vi "Read Actual Position.vi"(4 "error in (no error)":errorcluster, 6 "Axis (1)":i32=1 min=1 max=3, 7 "VISA resource name":refnum<visa-resource-name>) -> (0 "error out":errorcluster, 2 "Position (units)":dbl format="%.6g", 3 "VISA resource name out":refnum<visa-resource-name>)   [LabVIEW 2011, in "Newport ESP301.lvlib"]
doc: "Reads the current position.\nIt returns the instantaneous real position of the specified axis."
uses:
  Newport ESP301.lvlib
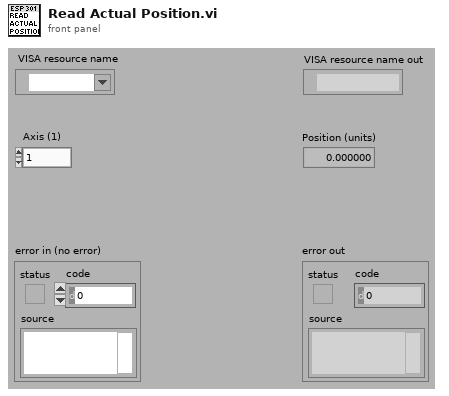
[diagram p1: front panel]
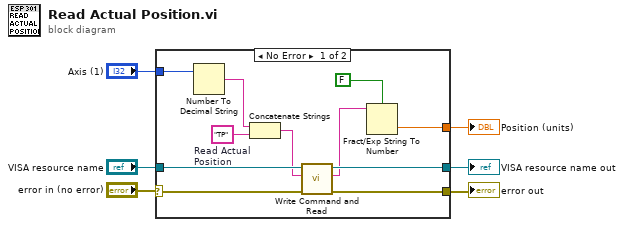
[diagram p0: block diagram]
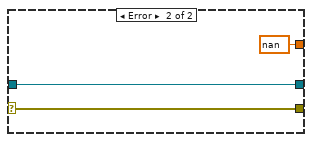
[diagram p2: hidden frame]
diagram:
  n1 = case shown="No Error" "error in (no error)" {
    selector: "error in (no error)" -> [w14 w20]
    tunnel: [w16 w20] -> w6
    tunnel: "VISA resource name" -> [w17 w19]
    tunnel: [w15 w19] -> w5
    tunnel: "Axis (1)" -> [w11 _]
    tunnel: [w8 nan] -> w1
    frame No Error {
      w13 = "TP"  # Read Actual Position
      n2 = Number To Decimal String(number=w11) -> (decimal integer string=w12:string)  [unwired: 1 in]
      n3 = Concatenate Strings(w12, w13) -> (w10:string)
      n4 = call "Write Command and Read.vi"("error in (no error)"=w14, "Command"=w10, "VISA resource name"=w17) -> ("error out"=w16:errorcluster, "Returned string"=w9:string, "VISA resource name out"=w15:refnum<visa-resource-name>)  [unwired: 4 in]
      n5 = Fract/Exp String To Number(use system decimal point (T)=FALSE ("utiliser le séparateur décimal du système (V)"), string=w9) -> (number=w8:dbl)  [unwired: 2 in, 1 out]
    }
    frame Error {
    }
  }
  "error out" <- w6
  "VISA resource name out" <- w5
  "Position (units)" <- w1
